vi "RBF Graph.vi"(4 "STD":dbl, 5 "Limit":cluster{"upper limit":dbl, "lower limit":dbl}={"upper limit"=0.3, "lower limit"=0.0} {"lower limit" format="%#_13g"; "upper limit" format="%#_13g"}, 6 "RBF Number":i32, 7 "RBF Weights":dbl[](array[numeric]), 8 "Scale":dbl format="%#_13g", 9 "x_f":dbl, 10 "x_0":dbl, 11 "Sample Number":i32) -> (3 "XY Graph":cluster{dbl[], dbl[]}[](array[cluster]))   [LabVIEW 2021]
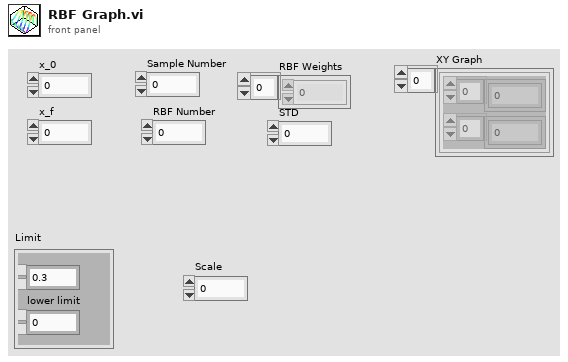
[diagram p1: front panel]
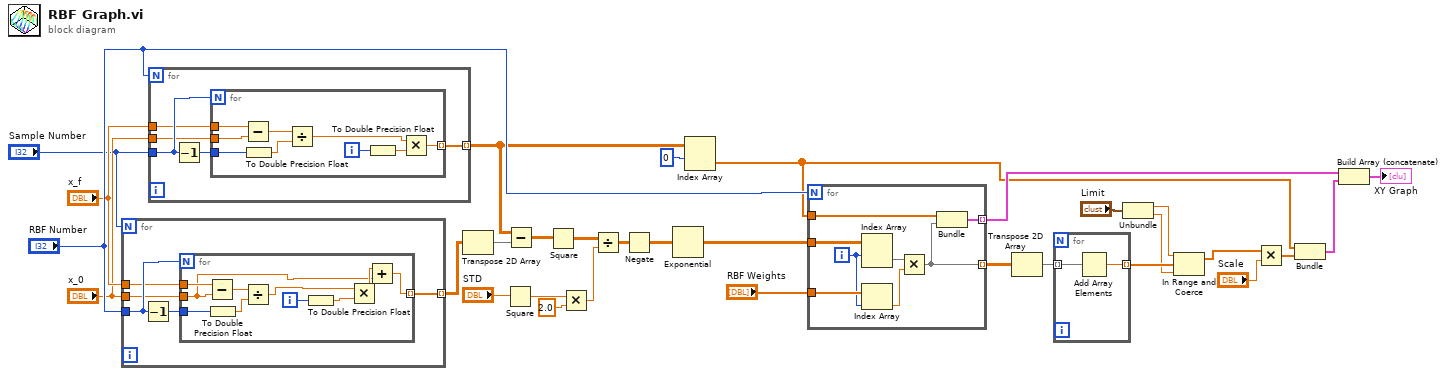
[diagram p0: block diagram]
diagram:
  n1 = for {
    N: "Sample Number" -> [_]
    tunnel: [w35] -> w18 mode=indexing
    tunnel: "RBF Number" -> [w34]
    tunnel: "x_f" -> [w33]
    tunnel: "x_0" -> [w32]
    n2 = Decrement(x=w34) -> (x-1=w36:i32)
    n3 = for {
      N: w34 -> [_]
      tunnel: w33 -> [w46]
      tunnel: w32 -> [w37]
      tunnel: [w39] -> w35 mode=indexing
      tunnel: w36 -> [w44]
      i -> [w42]
      n4 = Subtract(x=w46, y=w37) -> (x-y=w45:dbl)
      n5 = To Double Precision Float(number=w44) -> (double precision float=w43:dbl)
      n6 = Divide(x=w45, y=w43) -> (x/y=w40:dbl)
      n7 = To Double Precision Float(number=w42) -> (double precision float=w41:dbl)
      n8 = Multiply(x=w40, y=w41) -> (x*y=w38:dbl)
      n9 = Add(x=w38, y=w37) -> (x+y=w39:dbl)
    }
  }
  n10 = for {
    N: "RBF Number" -> [_]
    tunnel: [w50] -> w12 mode=indexing
    tunnel: "Sample Number" -> [w49]
    tunnel: "x_f" -> [w48]
    tunnel: "x_0" -> [w47]
    n11 = Decrement(x=w49) -> (x-1=w51:i32)
    n12 = for {
      N: w49 -> [_]
      tunnel: w48 -> [w60]
      tunnel: w47 -> [w58]
      tunnel: [w59] -> w50 mode=indexing
      tunnel: w51 -> [w55]
      i -> [w52]
      n13 = Subtract(x=w60, y=w58) -> (x-y=w57:dbl)
      n14 = To Double Precision Float(number=w55) -> (double precision float=w54:dbl)
      n15 = Divide(x=w57, y=w54) -> (x/y=w56:dbl)
      n16 = To Double Precision Float(number=w52) -> (double precision float=w53:dbl)
      n17 = Multiply(x=w56, y=w53) -> (x*y=w59:dbl)
    }
  }
  n18 = Transpose 2D Array(2D array=w18) -> (transposed array=w17:dbl[][])
  n19 = Square(x="STD") -> (x^2=w27:dbl)
  n20 = Subtract(x=w12, y=w17) -> (x-y=w23:dbl[][])
  n21 = Square(x=w23) -> (x^2=w22:dbl[][])
  n22 = Multiply(x=w27, y=2.0) -> (x*y=w30:dbl)
  n23 = Divide(x=w22, y=w30) -> (x/y=w21:dbl[][])
  n24 = Negate(x=w21) -> (-x=w20:dbl[][])
  n25 = Exponential(1:w20) -> (0:w9:dbl[][])
  n26 = Index Array(array=w12, index (row)=0) -> (element=w10:dbl[])  [unwired: 1 in]
  n27 = for {
    N: "RBF Number" -> [_]
    tunnel: w9 -> [w68]
    tunnel: [w67] -> w15 mode=indexing
    tunnel: "RBF Weights" -> [w66]
    tunnel: w10 -> [w62]
    tunnel: [w61] -> w8 mode=indexing
    i -> [w65]
    n28 = Index Array(array=w68, index (row)=w65) -> (element=w63:dbl[])  [unwired: 1 in]
    n29 = Index Array(array=w66, index=w65) -> (element=w64:dbl)
    n30 = Multiply(x=w63, y=w64) -> (x*y=w61:dbl[])
    n31 = Bundle(w62, w61) -> (w67:cluster{dbl[], dbl[]})  [unwired: 1 in]
  }
  n32 = Transpose 2D Array(2D array=w8) -> (transposed array=w16:dbl[][])
  n33 = for {
    tunnel: w16 -> [w70] mode=indexing
    tunnel: [w69] -> w7 mode=indexing
    n34 = Add Array Elements(numeric array=w70) -> (sum=w69:dbl)
  }
  n35 = Unbundle("Limit") -> ("upper limit"=w2:dbl, "lower limit"=w1:dbl)
  n36 = In Range and Coerce(upper limit=w2, x=w7, lower limit=w1) -> (coerced(x)=w6:dbl[])  [unwired: 1 out]
  n37 = Multiply(x=w6, y="Scale") -> (x*y=w5:dbl[])
  n38 = Bundle(w10, w5) -> (w13:cluster{dbl[], dbl[]})  [unwired: 1 in]
  n39 = Build Array (concatenate)(w15, w13) -> (→"XY Graph":cluster{dbl[], dbl[]}[])
